vi "Gage_to_labview_error.vi"(9 "Error In":errorcluster, 10 "GaGe Error Number":i32, 11 "Handle Cluster":T1) -> (0 "Error Out":errorcluster)   [LabVIEW 2015]
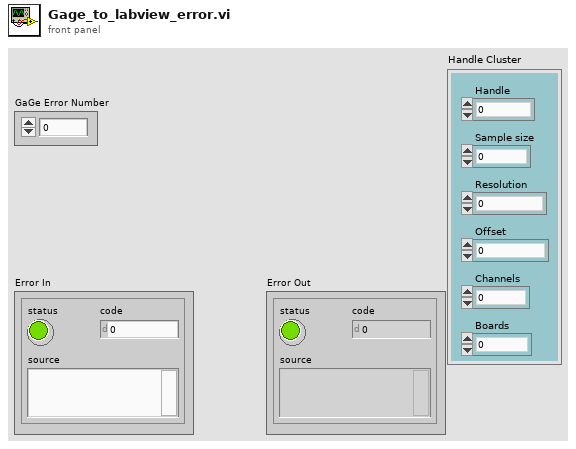
[diagram p1: front panel]
types:
  T1 = cluster{"Handle":u32, "Sample size":u32, "Resolution":i32, "Offset":i32, "Channels":u32, "Boards":u32}
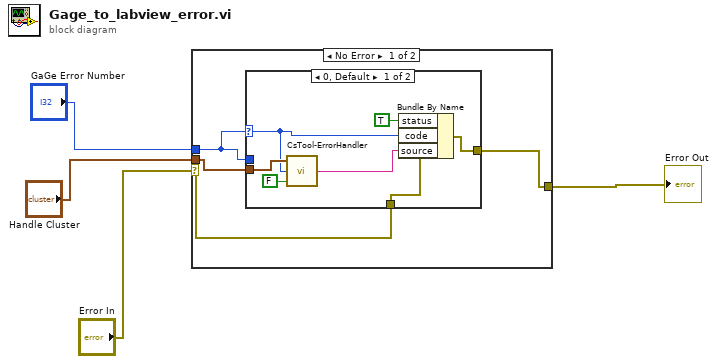
[diagram p0: block diagram]
diagram:
  n1 = case shown="No Error" "Error In" {
    selector: "Error In" -> [w8 w17]
    tunnel: [w7 w17] -> w3
    tunnel: "GaGe Error Number" -> [w6 _]
    tunnel: "Handle Cluster" -> [w5 _]
    frame No Error {
      n2 = case shown="0, Default" w6 {
        selector: w6 -> [w11 _]
        tunnel: w8 -> [w14 w16]
        tunnel: [w13 w16] -> w7
        tunnel: w6 -> [_ _]
        tunnel: w5 -> [w12 _]
        frame 0, Default {
          n3 = call <userlib>:"CsTool-ErrorHandler.vi"("StopOnError (true)"=FALSE, "Error Code"=w11, "Handle Cluster"=w12) -> ("Error String"=w10:string)
          n4 = Bundle By Name(cluster=w14, "status"=TRUE, "code"=w11, "source"=w10) -> (w13:errorcluster)
        }
        frame 1 {
        }
      }
    }
    frame Error {
    }
  }
  "Error Out" <- w3
